vi "试验配置信息.vi"() -> ()   [LabVIEW 2010]
panel:
  in  "LAN选择？":bool
  in  "RS485选择？":bool
  in  "RS232选择？":bool
  in  "CAN选择？":bool
  in  "AD输入选择？":bool
  in  "DSP输入选择？":bool
  in  "数字量输出选择？":bool
  in  "数字量输入选择？":bool
  in  "自测LAN路数":i32
  in  "自测项数":i32
  in  "自测类数":i32
  in  "自测AI_DSP路数":i32
  in  "自测485路数":i32
  in  "自测RS232路数":i32
  in  "自测CAN路数":i32
  in  "自测AI_AD路数":i32
  in  "自测DO路数":i32
  in  "自测DI路数":i32
  in  "报告编号":string
  in  "测试地点":string
  in  "测试人员":string
  in  "控制板编号":string
  in  "控制板类型":string
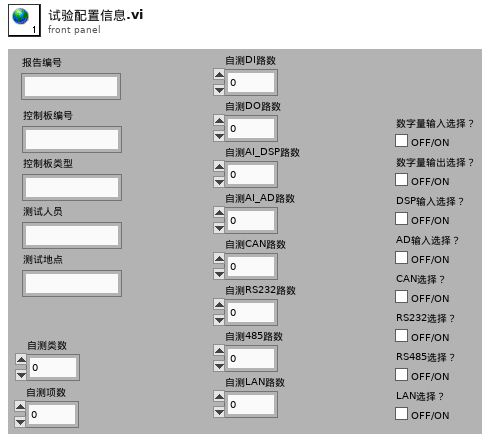
[diagram p1: front panel]
diagram:
